vi "Angle_around_X_axis.vi"(1 "gx":i32, 2 "dt":dbl=0.1) -> (0 "Angle around the X-axis (*pitch)":dbl)   [LabVIEW 2015]
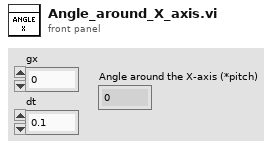
[diagram p1: front panel]
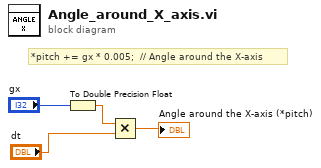
[diagram p0: block diagram]
diagram:
  # "*pitch += gx * 0.005;  // Angle around the X-axis"
  n1 = To Double Precision Float(number="gx") -> (double precision float=w1:dbl)
  n2 = Multiply(x=w1, y="dt") -> (x*y=→"Angle around the X-axis (*pitch)":dbl)
